vi "Get Timestamp.vi"(8 "error in (no error)":errorcluster, 10 "Offset":i32, 11 "JSON":string) -> (0 "error out":errorcluster, 1 "Timestamp":timestamp, 2 "Offset past match":i32)   [LabVIEW 2013, in "JSONtext.lvlib"]
uses:
  JSONtext.lvlib
  Advance past String.vi
  support/Strip Quotes and Unescape.vi
  Get Number Text.vi
  Advance past Number.vi
  Parsing Error.vi
  support/Unescape JSON string.vi
  support/JSONtext support.lvlib
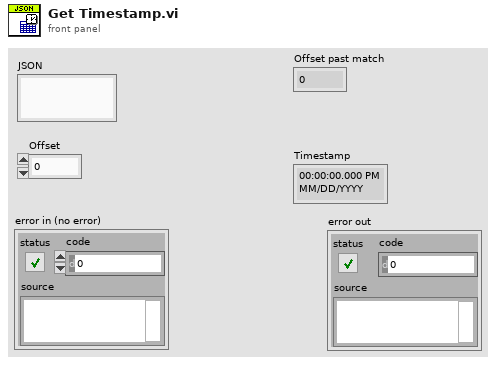
[diagram p1: front panel]
types:
  T1 = typedef "JSONtext.lvlib/Parsing State.ctl" = enum16{"Parser Error", "Object", "Array", "String", "Number/Other", "Leading Whitespace", "Object end", "Array end", "Value end"}
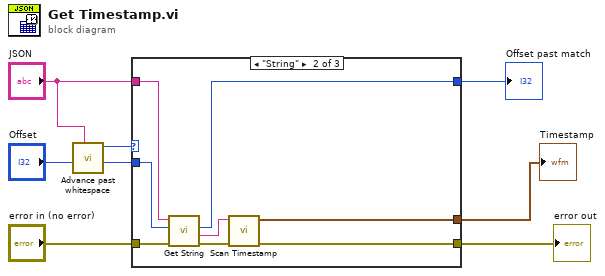
[diagram p0: block diagram]
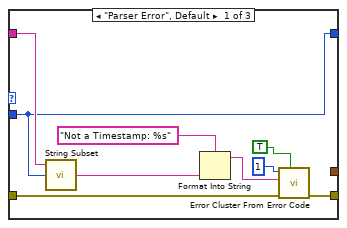
[diagram p2: hidden frame]
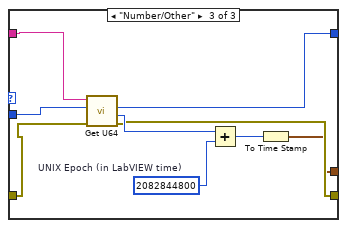
[diagram p3: hidden frame]
diagram:
  n1 = call "Advance past whitespace.vi"("JSON"="JSON", "Offset"="Offset") -> ("Offset of first non-whitespace"=w2:i32, "Parser State"=w1:T1)  [unwired: 8 in]
  n2 = case shown="\"String\"" w1 {
    tunnel: "error in (no error)" -> [w16 w25 w29]
    tunnel: [_ w22 w27] -> w7
    tunnel: [w17 w21 w28] -> w6
    tunnel: [w9 w20 w26] -> w5
    tunnel: "JSON" -> [w11 w19 w34]
    tunnel: w2 -> [w9 w18 w33]
    frame "Parser Error", Default {
      n3 = call "String Subset.vi"("Start offset"=w9, "JSON"=w11) -> ("substring"=w10:string)  [unwired: 3 in]
      n4 = Format Into String(format string="Not a Timestamp: %s", w10) -> (resulting string=w12:string)  [unwired: 2 in, 1 out]
      n5 = call <vilib>:"Error Cluster From Error Code.vi"("show call chain? (False)"=TRUE, "error in (no error)"=w16, "error message (\"\")"=w12, "error code (0)"=1) -> ("error out"=w17:errorcluster)  [unwired: 5 in]
    }
    frame "String" {
      n6 = call "Get String.vi"("error in (no error)"=w25, "Offset"=w18, "JSON"=w19) -> ("error out"=w24:errorcluster, "String"=w23:string, "Offset past match"=w20:i32)  [unwired: 6 in]
      n7 = call "Scan Timestamp.vi"("error in (no error)"=w24, "String"=w23) -> ("error out"=w21:errorcluster, "Timestamp"=w22:timestamp)  [unwired: 8 in]
    }
    frame "Number/Other" {
      w32 = i64 2082844800  # UNIX Epoch (in LabVIEW time)
      n8 = call "Get U64.vi"("error in (no error)"=w29, "Offset"=w33, "JSON"=w34) -> ("error out"=w28:errorcluster, "Number"=w30:u64, "Offset past match"=w26:i32)  [unwired: 6 in]
      n9 = Add(x=w30, y=w32) -> (x+y=w31:u64)
      n10 = To Time Stamp(1:w31) -> (0:w27:timestamp)
    }
  }
  "error out" <- w6
  "Offset past match" <- w5
  "Timestamp" <- w7
